vi "ReadLowTemp.vi"(7 "error in (no error)":errorcluster) -> (0 "error out":errorcluster, 1 "CurrentTemp(LowChamber)":dbl, 2 "CurrentTemp(LowChamber)":string)   [LabVIEW 2017, in "Thermal Shock.lvlib"]
uses:
  Thermal Shock.lvlib
  <vilib>/Instr/_visa.llb/VISA Configure Serial Port (Instr).vi
panel:
  in  "Read Low Chamber!":bool
  out "LowChamberSetPoint":dbl
  in  "Stop":bool
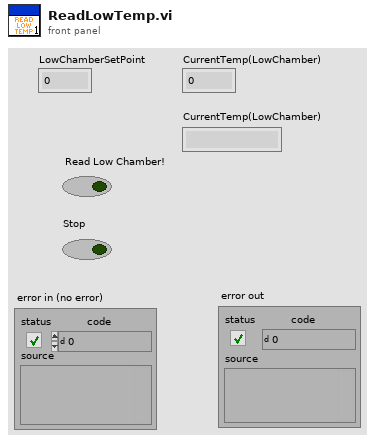
[diagram p1: front panel]
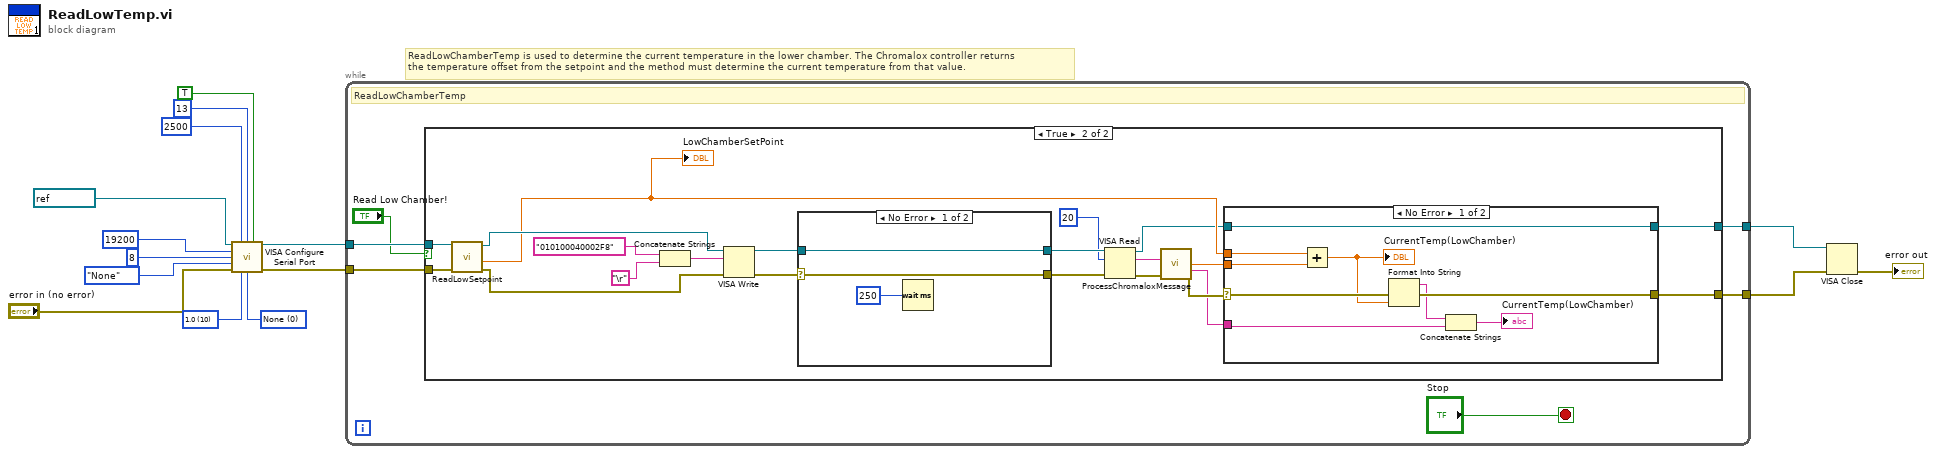
[diagram p0: block diagram]
diagram:
  w7 = u16 0 items=["None", "XON/XOFF", "RTS/CTS", "XON/XOFF & RTS/CTS", "DTR/DSR", "XON/XOFF & DTR/DSR"] ("flow control (0:none)")
  w9 = u16 10 items=["1.0"=10, "1.5"=15, "2.0"=20] ("stop bits (10: 1 bit)")
  # "ReadLowChamberTemp is used to determine the current temperature in the lower chamber. The Chromalox controller returns \nthe temperature offset from the setpoint and the method must determine the current temperature from that value."
  n1 = call-poly "VISA Configure Serial Port"("VISA resource name"=refnum<visa-resource-name> "COM1", "timeout (10sec)"=2500, "termination char\n(0xA = '\\n' = LF)"=u8 13, "Enable Termination\nChar (T)"=TRUE, "baud rate (9600)"=19200, "data bits (8)"=u16 8, "parity (0:none)"=enum16{"None", "Odd", "Even", "Mark", "Space"}."None", "error in (no error)"="error in (no error)", "stop bits (10: 1 bit)"=w9, "flow control (0:none)"=w7) -> ("VISA resource name out"=w5:refnum<visa-resource-name>, "error out"=w4:errorcluster)  [unwired: 4 in]
  n2 = while {
    tunnel: w5 -> [w20]
    tunnel: w4 -> [w19]
    tunnel: [w18] -> w3
    tunnel: [w17] -> w2
    stop <- "Stop" stop-if-true
    # "ReadLowChamberTemp"
    n3 = case shown="True" "Read Low Chamber!" {
      tunnel: w20 -> [w23 w41]
      tunnel: w19 -> [w22 w40]
      tunnel: [w22 w28] -> w18
      tunnel: [w23 w26] -> w17
      frame False {
      }
      frame True {
        n4 = call "ReadLowSetpoint.vi"("error in (no error)"=w40, "VISA resource name"=w41) -> ("error out"=w38:errorcluster, "LowChamberSetPoint"=w29:dbl, "VISA resource name out"=w39:refnum<visa-resource-name>)  [unwired: 6 in, 1 out]
        "LowChamberSetPoint" <- w29
        n5 = Concatenate Strings("010100040002F8", "\r") -> (w42:string)
        n6 = VISA Write(VISA resource name=w39, write buffer=w42, error in (no error)=w38) -> (VISA resource name out=w36:refnum<visa-resource-name>, error out=w37:errorcluster)  [unwired: 1 out]
        n7 = case shown="No Error" w37 {
          selector: w37 -> [w58 w59]
          tunnel: w36 -> [w57 w60]
          tunnel: [w58 w59] -> w34
          tunnel: [w57 w60] -> w35
          frame No Error {
            n8 = Wait (ms)(milliseconds to wait=250) -> ()  [unwired: 1 out]
          }
          frame Error {
          }
        }
        n9 = VISA Read(VISA resource name=w35, byte count=20, error in (no error)=w34) -> (VISA resource name out=w27:refnum<visa-resource-name>, read buffer=w32:string, error out=w31:errorcluster)  [unwired: 1 out]
        n10 = call "ProcessChromaloxMessage.vi"("Chromalox Message"=w32, "error in (no error)"=w31) -> ("Reading"=w24:dbl, "Units"=w25:string, "error out"=w30:errorcluster)  [unwired: 10 in, 1 out]
        n11 = case shown="No Error" w30 {
          selector: w30 -> [w52 w55]
          tunnel: w29 -> [w46 _]
          tunnel: [w51 w55] -> w28
          tunnel: w27 -> [w53 w54]
          tunnel: [w53 w54] -> w26
          tunnel: w25 -> [w48 _]
          tunnel: w24 -> [w45 _]
          frame No Error {
            n12 = Add(x=w46, y=w45) -> (x+y=w50:dbl)
            "CurrentTemp(LowChamber)" <- w50
            n13 = Format Into String(error in=w52, w50) -> (resulting string=w49:string, error out=w51:errorcluster)  [unwired: 2 in]
            n14 = Concatenate Strings(w49, w48) -> (→"CurrentTemp(LowChamber)":string)
          }
          frame Error {
          }
        }
      }
    }
  }
  n15 = VISA Close(VISA resource name=w2, error in (no error)=w3) -> (error out=→"error out":errorcluster)
